vi "niFpgaClipTempStateGlobal.vi"() -> ()   [LabVIEW 2017]
uses:
  <vilib>/rvi/ClientSDK/Clip/niFpgaClipItemState.ctl
  <vilib>/rvi/Clip/Clip_types/nirviClip_CLIPClockConnection.ctl
  <vilib>/rvi/Clip/Clip_types/nirviClip_CLIPClock.ctl
  <resource>/RVI/StockIO/private/niLVFPGA_CLIP_ModGen/niLVFPGA_CLIP_typedef_CLIPSignalDirection.ctl
  <vilib>/rvi/Clip/Clip_types/nirviClip_FpgaClock.ctl
  <vilib>/rvi/Clip/Clip_types/nirviClip_CLIPGeneric.ctl
  <vilib>/rvi/Clip/Clip_types/nirviClip_CLIPInstanceSignal.ctl
  <vilib>/fxp/LVFixedPointRepBitsTypeDef.ctl
  <resource>/RVI/StockIO/private/niLVFPGA_CLIP_ModGen/niLVFPGA_CLIP_typedef_CLIPSignalInterfaceType.ctl
  <resource>/RVI/StockIO/private/niLVFPGA_CLIP_ModGen/niLVFPGA_CLIP_typedef_CLIPSignalType.ctl
  <resource>/RVI/StockIO/private/topModGenUtilities/niFpgaCompilerSettings.ctl
  <vilib>/rvi/ClientSDK/Core/CompilationInfo/niFpgaCompilationToolVersion_compiler.ctl
  <vilib>/rvi/IPIntegrationNode/IPINode_Typedef/niFpgaIPINodeXilinxProc.ctl
  <vilib>/rvi/IPIntegrationNode/IPINode_Typedef/niFpgaIPINodeOwningTarget.ctl
panel:
  in  "Clip Configuration":T1={"Name"="", "Extended Name"="", "Glyph Path"=path "", "Extended Config String"="", "Socketed CLIP?"=FALSE, "Socket Selection"="", "Declaration Category"="", "Declaration Name"="", "Clock Connections"=[], "Socket Specific Compile Signature"="", "Generics"=[], "Instance Signal Info"=[], "Temp Work Dir"=path "", "Compiler Settings"={"Constraint File Type"="", "Compiler"=enum."Xilinx ISE", "Core Config File Type"="", "Xilinx Process"=enum."Fuse", "OwningTarget"=enum."IseTarget"}}
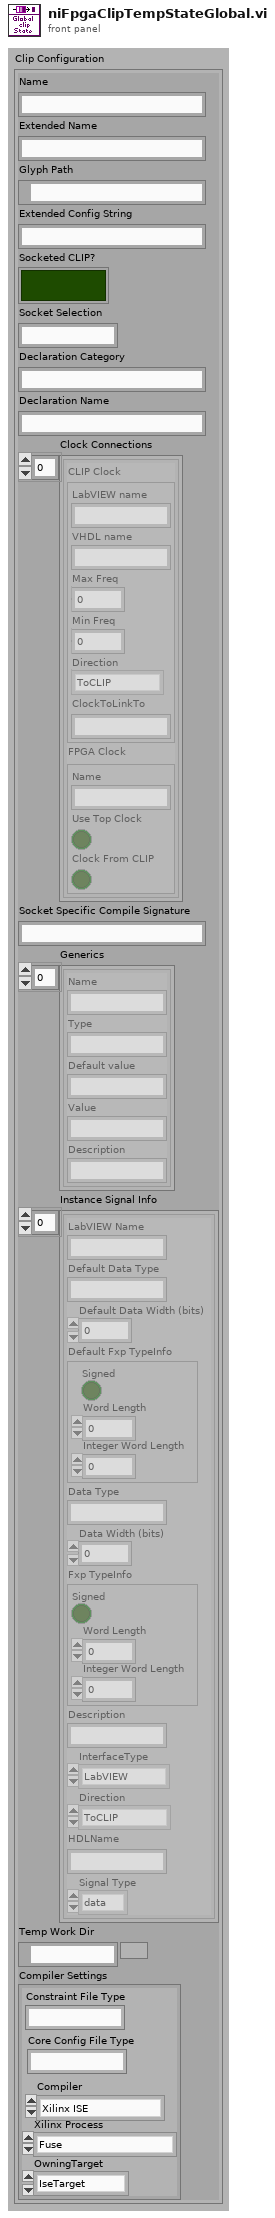
[diagram p1: front panel]
types:
  T1 = typedef "niFpgaClipItemState.ctl" = cluster{"Name":string, "Extended Name":string, "Glyph Path":path, "Extended Config String":string, "Socketed CLIP?":bool, "Socket Selection":string, "Declaration Category":string, "Declaration Name":string, "Clock Connections":T2[], "Socket Specific Compile Signature":string, "Generics":T6[], "Instance Signal Info":T7[], "Temp Work Dir":path, "Compiler Settings":T11}
  T2 = typedef "nirviClip_CLIPClockConnection.ctl" = cluster{"CLIP Clock":T3, "FPGA Clock":T5}
  T3 = typedef "nirviClip_CLIPClock.ctl" = cluster{"LabVIEW name":string, "VHDL name":string, "Max Freq":dbl, "Min Freq":dbl, "Direction":T4, "ClockToLinkTo":string}
  T4 = typedef "niLVFPGA_CLIP_typedef_CLIPSignalDirection.ctl" = enum16{"ToCLIP", "FromCLIP", "Bidirectional"}
  T5 = typedef "nirviClip_FpgaClock.ctl" = cluster{"Name":string, "Use Top Clock":bool, "Clock From CLIP":bool}
  T6 = typedef "nirviClip_CLIPGeneric.ctl" = cluster{"Name":string, "Type":string, "Default value":string, "Value":string, "Description":string}
  T7 = typedef "nirviClip_CLIPInstanceSignal.ctl" = cluster{"LabVIEW Name":string, "Default Data Type":string, "Default Data Width (bits)":u32, "Default Fxp TypeInfo":cluster{"Signed":bool, "Word Length":u32, "Integer Word Length":i32}, "Data Type":string, "Data Width (bits)":u32, "Fxp TypeInfo":T8, "Description":string, "InterfaceType":T9, "Direction":T4, "HDLName":string, "Signal Type":T10}
  T8 = typedef "LVFixedPointRepBitsTypeDef.ctl" = cluster{"Signed":bool, "Word Length":u32, "Integer Word Length":i32}
  T9 = typedef "niLVFPGA_CLIP_typedef_CLIPSignalInterfaceType.ctl" = enum16{"LabVIEW", "Socket", "Fabric"}
  T10 = typedef "niLVFPGA_CLIP_typedef_CLIPSignalType.ctl" = enum16{"data", "clock", "socketed_data", "socketed_clock", "reset", "clock status", "clock gate"}
  T11 = typedef "niFpgaCompilerSettings.ctl" = cluster{"Constraint File Type":string, "Compiler":T12, "Core Config File Type":string, "Xilinx Process":T13, "OwningTarget":T14}
  T12 = typedef "niFpgaCompilationToolVersion_compiler.ctl" = enum16{"Xilinx ISE", "Xilinx Vivado"}
  T13 = typedef "niFpgaIPINodeXilinxProc.ctl" = enum16{"WriteVHDL_Netlist", "WriteVHDL_DCP", "GenerateTarget", "Fuse", "Coregen", "Netgen", "Xst_Elaborate", "NGCBuild", "Xelab", "Vivado_Elaborate"}
  T14 = typedef "niFpgaIPINodeOwningTarget.ctl" = enum8{"MyComputer", "VivadoTarget", "IseTarget"}
diagram:
